vi "Receive Dashboard Packet.vi"(7 "connection ID":refnum<k16>) -> ()   [LabVIEW 2015]
uses:
  Common Code/Dashboard Communication/Dashboard Control Data.ctl
  Common Code/Encoder Control.ctl
  Common Code/Drivetrain Settings.ctl
  Common Code/Goal Vision Packet.ctl
  Common Code/Dashboard Drivetrain Command.ctl
  Common Code/Drivetrain Vision.ctl
  Common Code/Ball Tracking Command Cluster.ctl
  Common Code/Ball Vision Packet.ctl
  Common Code/Tracking Mode.ctl
  Common Code/Intake Presets.ctl
  Common Code/Drivetrain Output Range.ctl
  Common Code/IntakeEcoderControl.ctl
  Common Code/Climb Presets.ctl
  Common Code/Enabled Systems.ctl
  Common Code/Autonomous Presets.ctl
  Common Code/Auto Shift Cluster.ctl
  Common Code/Catapult/Catapult Presets.ctl
  Common Code/Manipulator Control Indexes.ctl
  Common Code/Driver Control Indexes.ctl
  Common Code/Driver Control Label.ctl
  Common Code/Manipulator Control Label.ctl
  Robot Global Data.vi
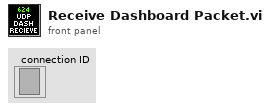
[diagram p1: front panel]
types:
  T1 = typedef "Dashboard Control Data.ctl" = cluster{"Encoder Control":T2, "Steer PID output":cluster{"output high":dbl, "output low":dbl}, " Steer PID gains":cluster{"proportional gain (Kc)":dbl, "integral time (Ti, min)":dbl, "derivative time (Td, min)":dbl}, "Drivetrain Settings":T3, "Vision Packet":T4, "Dashboard Drivetrain Command":T5, "Info/Command Cluster":T7, "Ball Vision Packet":T8, "Intake Presets":T10, "Intake Encoder Control":T12, "Climb Presets":T13, "Goal Output Range":cluster{"output high":dbl, "output low":dbl}, "Enabled Systems":T14, "Auton Presets":T15, "Pressure M":dbl, "Pressure B":dbl, "Vision Timeout":dbl, "Auto-Shift":T16, "Catapult Setpoints":T17, "Manipulator Control Indexes":T18, "Driver Control Indexes":T19, "Driver Label":T20, "Manipulator Label":T21}
  T2 = typedef "Encoder Control.ctl" = cluster{"Right Tick Constant":dbl, "Left Tick Constant":dbl, "Reset?":bool, "Y Dist":cluster{"PID gains":cluster{"proportional gain (Kc)":dbl, "integral time (Ti, min)":dbl, "derivative time (Td, min)":dbl}}, "Y Stop Thresh":dbl, "Y Stop Speed":dbl}
  T3 = typedef "Drivetrain Settings.ctl" = cluster{"Gyro Tolerance":dbl, "Throttle Ramp (ms)":dbl, "Kv":dbl, "Ka":dbl, "Feed Forward P":dbl, "Feed Forward D":dbl, "Goal Vision PID gains":cluster{"proportional gain (Kc)":dbl, "integral time (Ti, min)":dbl, "derivative time (Td, min)":dbl}, "Goal Detection Window":dbl, "Creep Rate":dbl, "Vision Throttle Threshold":dbl, "Min Turn Output":dbl, "Left Batter Angle":dbl, "Right Batter Angle":dbl}
  T4 = typedef "Goal Vision Packet.ctl" = cluster{"Distance":dbl, "Center X":dbl, "Center Y":dbl, "Found Target?":bool, "Robot Center":dbl, "Angle":dbl}
  T5 = typedef "Dashboard Drivetrain Command.ctl" = cluster{"Drivetrain Vision":T6}
  T6 = typedef "Drivetrain Vision.ctl" = cluster{"Goal Window":dbl, "Ball Window":dbl}
  T7 = typedef "Ball Tracking Command Cluster.ctl" = cluster{"Distance to Ball":dbl, "Desired Angle":dbl, "Command":enum16{"Turn to Ball", "Turn to Angle", "Get Distance"}, "Pixels from Center":dbl}
  T8 = typedef "Ball Vision Packet.ctl" = cluster{"Ball Detected?":bool, "Distance to Ball":dbl, "Desired Angle":dbl, "Pixels from Center":dbl, "Tracking mode":T9}
  T9 = typedef "Tracking Mode.ctl" = enum16{"Turn to Ball", "Turn to Angle"}
  T10 = typedef "Intake Presets.ctl" = cluster{"Intake Speed":dbl, "Outake Speed":dbl, "Low Height":dbl, "Half Height":dbl, "High Idle Height":dbl, "Angle Speed":dbl, "Angle Tolerance":dbl, "Encoder Scale":dbl, "Load Height":dbl, "Output Range":T11, "Rotation Power Max/Min":dbl, "MaxCurrent":dbl, "Intake Trip Time":dbl, "Idle Height":dbl, "Max Height":dbl, "Reset Encoders?":bool, "PID gains":cluster{"proportional gain (Kc)":dbl, "integral time (Ti, min)":dbl, "derivative time (Td, min)":dbl}, "Intake Stop Delay":u32, "Settle Time":dbl, "Settle Wait Time":dbl, "Pull Up Delay":dbl}
  T11 = typedef "Drivetrain Output Range.ctl" = cluster{"output high":dbl, "output low":dbl}
  T12 = typedef "IntakeEcoderControl.ctl" = cluster{"Arm Tick Constant":dbl, "Reset?":bool, "Y Dist":cluster{"PID gains":cluster{"proportional gain (Kc)":dbl, "integral time (Ti, min)":dbl, "derivative time (Td, min)":dbl}}, "Y Stop Thresh":dbl, "Y Stop Speed":dbl}
  T13 = typedef "Climb Presets.ctl" = cluster{"Pull Power":dbl, "Extend Power":dbl}
  T14 = typedef "Enabled Systems.ctl" = cluster{"Shoot":bool, "Intake":bool, "DT":bool, "Gyro":bool, "100ms":bool, "US":bool}
  T15 = typedef "Autonomous Presets.ctl" = cluster{"Pitch Limit":dbl, "Roll Limit":dbl, "Start Position":dbl, "Cross Position":dbl}
  T16 = typedef "Auto Shift Cluster.ctl" = cluster{"Delay":dbl, "Speed Thresh":dbl, "Upshift Accel":dbl, "Upshift Throttle":dbl, "Upshift Throttle Accel":dbl, "Downshift Throttle":dbl, "Downshift Throttle Accel":dbl, "Pressure Threshold":dbl}
  T17 = typedef "Catapult Presets.ctl" = cluster{"Intake Danger Height":dbl, "Ball Security Delay ":dbl, "High PSI Minimum":dbl, "Shot Finish Delay":dbl, "Low PSI Minimum":dbl, "Idle Ball Security Wait ":dbl}
  T18 = typedef "Manipulator Control Indexes.ctl" = cluster{"High Pressure Shot":dbl, "Manual Climb Mode":dbl, "Auto Climb Mode":dbl, "Eject":dbl, "Intake":dbl, "Manual/Auto Toggle":dbl, "Re-seat":dbl, "Intake Down":dbl}
  T19 = typedef "Driver Control Indexes.ctl" = cluster{"Outer Shot":dbl, "Batter Shot":dbl, "Shoot":dbl, "Climb":dbl, "Flash Light":dbl}
  T20 = typedef "Driver Control Label.ctl" = cluster{"Outer Shot":string, "Batter Shot":string, "Shoot":string, "Climb":string, "Flashlight":string}
  T21 = typedef "Manipulator Control Label.ctl" = cluster{"High Pressure Shot":string, "Manual Climb Mode":string, "Auto Climb Mode":string, "Eject":string, "Intake":string, "Manual/Auto Toggle":string, "Re-seat":string, "Intake Down":string}
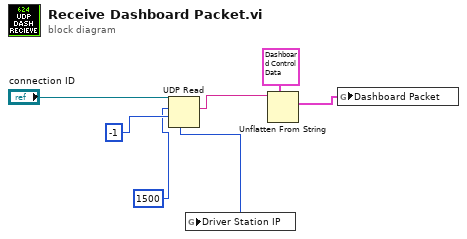
[diagram p0: block diagram]
diagram:
  n1 = UDP Read(connection ID="connection ID", max size (548)=1500, timeout ms (25000)=-1) -> (data out=w4:string, 6:w3:u32)  [unwired: 1 in, 3 out]
  n2 = global write "Robot Global Data.vi" "Driver Station IP"(w3) -> ()
  n3 = Unflatten From String(type=T1 {"Encoder Control"={"Right Tick Constant"=0.0, "Left Tick Constant"=0.0, "Reset?"=FALSE, "Y Dist"={"PID gains"={"proportional gain (Kc)"=0.0, "integral time (Ti, min)"=0.0, "derivative time (Td, min)"=0.0}}, "Y Stop Thresh"=0.0, "Y Stop Speed"=0.0}, "Steer PID output"={"output high"=0.0, "output low"=0.0}, " Steer PID gains"={"proportional gain (Kc)"=0.0, "integral time (Ti, min)"=0.0, "derivative time (Td, min)"=0.0}, "Drivetrain Settings"={"Gyro Tolerance"=0.0, "Throttle Ramp (ms)"=0.0, "Kv"=0.0, "Ka"=0.0, "Feed Forward P"=0.0, "Feed Forward D"=0.0, "Goal Vision PID gains"={"proportional gain (Kc)"=0.0, "integral time (Ti, min)"=0.0, "derivative time (Td, min)"=0.0}, "Goal Detection Window"=0.0, "Creep Rate"=0.0, "Vision Throttle Threshold"=0.0, "Min Turn Output"=0.0, "Left Batter Angle"=0.0, "Right Batter Angle"=0.0}, "Vision Packet"={"Distance"=0.0, "Center X"=0.0, "Center Y"=0.0, "Found Target?"=FALSE, "Robot Center"=0.0, "Angle"=0.0}, "Dashboard Drivetrain Command"={"Drivetrain Vision"={"Goal Window"=0.0, "Ball Window"=0.0}}, "Info/Command Cluster"={"Distance to Ball"=0.0, "Desired Angle"=0.0, "Command"=enum."Turn to Ball", "Pixels from Center"=0.0}, "Ball Vision Packet"={"Ball Detected?"=FALSE, "Distance to Ball"=0.0, "Desired Angle"=0.0, "Pixels from Center"=0.0, "Tracking mode"=enum."Turn to Ball"}, "Intake Presets"={"Intake Speed"=0.0, "Outake Speed"=0.0, "Low Height"=0.0, "Half Height"=0.0, "High Idle Height"=0.0, "Angle Speed"=0.0, "Angle Tolerance"=0.0, "Encoder Scale"=0.0, "Load Height"=0.0, "Output Range"={"output high"=0.0, "output low"=0.0}, "Rotation Power Max/Min"=0.0, "MaxCurrent"=0.0, "Intake Trip Time"=0.0, "Idle Height"=0.0, "Max Height"=0.0, "Reset Encoders?"=FALSE, "PID gains"={"proportional gain (Kc)"=0.0, "integral time (Ti, min)"=0.0, "derivative time (Td, min)"=0.0}, "Intake Stop Delay"=0, "Settle Time"=0.0, "Settle Wait Time"=0.0, "Pull Up Delay"=0.0}, "Intake Encoder Control"={"Arm Tick Constant"=0.0, "Reset?"=FALSE, "Y Dist"={"PID gains"={"proportional gain (Kc)"=0.0, "integral time (Ti, min)"=0.0, "derivative time (Td, min)"=0.0}}, "Y Stop Thresh"=0.0, "Y Stop Speed"=0.0}, "Climb Presets"={"Pull Power"=0.0, "Extend Power"=0.0}, "Goal Output Range"={"output high"=0.0, "output low"=0.0}, "Enabled Systems"={"Shoot"=TRUE, "Intake"=TRUE, "DT"=TRUE, "Gyro"=TRUE, "100ms"=TRUE, "US"=TRUE}, "Auton Presets"={"Pitch Limit"=0.0, "Roll Limit"=0.0, "Start Position"=0.0, "Cross Position"=0.0}, "Pressure M"=0.0, "Pressure B"=0.0, "Vision Timeout"=0.0, "Auto-Shift"={"Delay"=0.0, "Speed Thresh"=0.0, "Upshift Accel"=0.0, "Upshift Throttle"=0.0, "Upshift Throttle Accel"=0.0, "Downshift Throttle"=0.0, "Downshift Throttle Accel"=0.0, "Pressure Threshold"=0.0}, "Catapult Setpoints"={"Intake Danger Height"=0.0, "Ball Security Delay "=0.0, "High PSI Minimum"=0.0, "Shot Finish Delay"=0.0, "Low PSI Minimum"=0.0, "Idle Ball Security Wait "=0.0}, "Manipulator Control Indexes"={"High Pressure Shot"=0.0, "Manual Climb Mode"=0.0, "Auto Climb Mode"=0.0, "Eject"=0.0, "Intake"=0.0, "Manual/Auto Toggle"=0.0, "Re-seat"=0.0, "Intake Down"=0.0}, "Driver Control Indexes"={"Outer Shot"=0.0, "Batter Shot"=0.0, "Shoot"=0.0, "Climb"=0.0, "Flash Light"=0.0}, "Driver Label"={"Outer Shot"="", "Batter Shot"="", "Shoot"="", "Climb"="", "Flashlight"=""}, "Manipulator Label"={"High Pressure Shot"="", "Manual Climb Mode"="", "Auto Climb Mode"="", "Eject"="", "Intake"="", "Manual/Auto Toggle"="", "Re-seat"="", "Intake Down"=""}} ("Dashboard Control Data"), binary string=w4) -> (value=w1:T1)  [unwired: 3 in, 2 out]
  n4 = global write "Robot Global Data.vi" "Dashboard Packet"(w1) -> ()
